vi "test_OneSessOnePinGroupOneInstrOneSiteReservation_CallNiDcPowerGetConnections1PinMConnections_ReturnsTwoConnections.vi"() -> (6 "pass":bool, 8 "result":string, 15 "error out":errorcluster)   [LabVIEW 2020, in "MeasurementServerTests.lvlib"]
uses:
  MeasurementServerTests.lvlib
  Runtime/Sessions/niDCPower Sessions/niDCPower Sessions.lvlib
  0bcc7825-b361-4d47-8536-1ed12f6e0935.vi
  Runtime/Measurements/Measurement Plugin Session Management V1/Session Reservation/Connection.ctl
  Runtime/Measurements/Measurement Plugin Session Management V1/Session Reservation/Session Reservation.lvclass
  Runtime/Sessions/niDCPower Sessions/Connection with Session.ctl
  Runtime/Sessions/niDCPower Sessions/Get Connections - 1Pin MConn.vi
panel:
  in  "error in":errorcluster
  # "Test assumes discovery service, pin map service, and session management service have already been started."
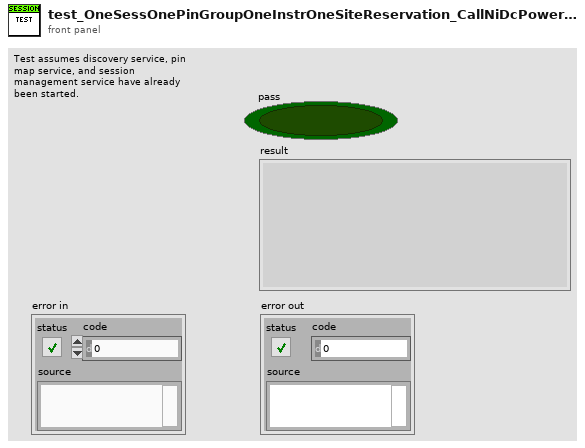
[diagram p1: front panel]
types:
  T1 = typedef "niDCPower Sessions.lvlib/Connection with Session.ctl" = cluster{"connection":T2, "session":refnum<k15>}
  T2 = typedef "Measurement Plugin Session Management V1.lvlib/Session Reservation.lvclass/Connection.ctl" = cluster{"pin or relay name":string, "site":i32, "instrument type id":string, "channel":string}
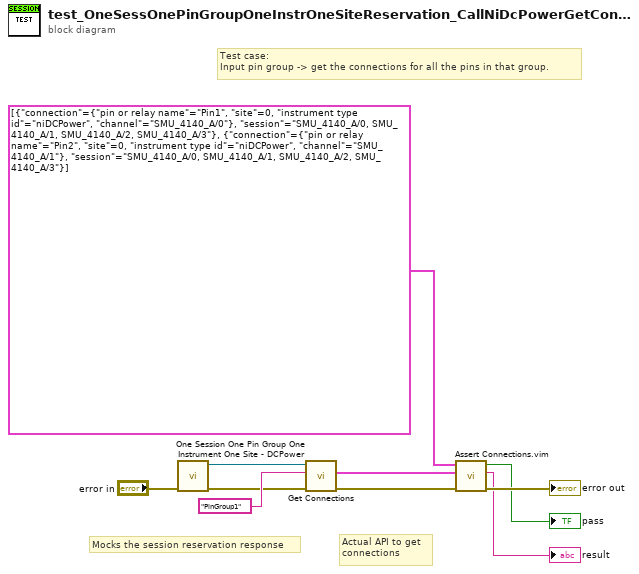
[diagram p0: block diagram]
diagram:
  # "Actual API to get\nconnections"
  # "Mocks the session reservation response"
  # "Test case:\nInput pin group -> get the connections for all the pins in that group."
  n1 = call "One Session One Pin Group One Instrument One Site - DCPower.vi"("error in"="error in") -> ("error out"=w1:errorcluster, "session reservation out"=w3:refnum<class "Session Reservation.lvclass">)  [unwired: 9 in]
  n2 = call-poly "Get Connections.vi"("error in"=w1, "pin or relay name"="PinGroup1", "session reservation in"=w3) -> ("error out"=w9:errorcluster, "connections"=w4:T1[])  [unwired: 6 in, 1 out]
  n3 = call "Assert Connections.vim"("error in"=w9, "actual connections"=w4, "expected connections"=T1[] [{"connection"={"pin or relay name"="Pin1", "site"=0, "instrument type id"="niDCPower", "channel"="SMU_4140_A/0"}, "session"="SMU_4140_A/0, SMU_4140_A/1, SMU_4140_A/2, SMU_4140_A/3"}, {"connection"={"pin or relay name"="Pin2", "site"=0, "instrument type id"="niDCPower", "channel"="SMU_4140_A/1"}, "session"="SMU_4140_A/0, SMU_4140_A/1, SMU_4140_A/2, SMU_4140_A/3"}] ("appended array")) -> ("error out"=→"error out":errorcluster, "result"=→"result":string, "pass"=→"pass":bool)  [unwired: 6 in]
